vi "GenNet Message Received.vi"(8 "error in":errorcluster, 10 "Message":variant, 11 "Module ID":i32=-1) -> (0 "error out":errorcluster)   [LabVIEW 2020, in "GenNet-Server.lvlib"]
doc: "Broadcasts a received <b>message</b> as variant datatype. The actual datatype (and decoding) of the variant depends on the GenNet Protocol being used.\n____\nHAMPEL SOFTWARE ENGINEERING v3.8.0 (2023-12-18 14:41)"
uses:
  GenNet-Server.lvlib
  GenNet Message Received Argument--cluster.ctl
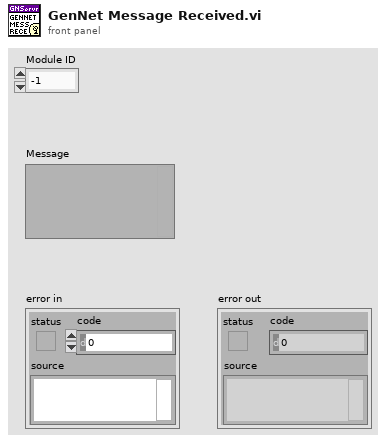
[diagram p1: front panel]
types:
  T1 = typedef "GenNet-Server.lvlib/GenNet Message Received Argument--cluster.ctl" = cluster{"Module ID":i32, "Message":variant}
  T2 = typedef "GenNet-Server.lvlib/Broadcast Events--cluster.ctl" = cluster{"Module Did Init":refnum<user-event>, "Status Updated":refnum<user-event>, "Error Reported":refnum<user-event>, "Module Did Stop":refnum<user-event>, "Update Module Execution Status":refnum<user-event>, "GenNet Message Received":refnum<user-event>}
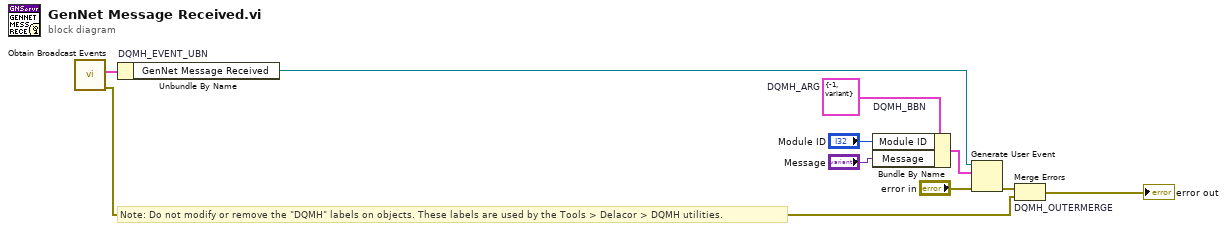
[diagram p0: block diagram]
diagram:
  w5 = T1 {"Module ID"=-1, "Message"=variant}  # DQMH_ARG
  # "Note: Do not modify or remove the \"DQMH\" labels on objects. These labels are used by the Tools > Delacor > DQMH utilities."
  n1 = call "Obtain Broadcast Events.vi"() -> ("error out"=w2:errorcluster, "GenNet-Server Broadcast Events"=w1:T2)  [unwired: 10 in]
  n2 = Unbundle By Name "DQMH_EVENT_UBN"(w1) -> ("GenNet Message Received"=w7:refnum<user-event>)
  n3 = Bundle By Name "DQMH_BBN"(cluster=w5, "Module ID"="Module ID", "Message"="Message") -> (w8:T1)
  n4 = Generate User Event(user event=w7, event data cluster=w8, error in="error in") -> (error out=w6:errorcluster)  [unwired: 1 in, 1 out]
  n5 = Merge Errors "DQMH_OUTERMERGE"(w6, w2) -> (→"error out":errorcluster)
